vi "Continuous Euler Angles.vi"() -> ()   [LabVIEW 2012]
uses:
  <vilib>/Platform/TimedLoop/XDataNode/timing_clust.ctl
  <vilib>/Platform/TimedLoop/XDataNode/nitl_modes.ctl
  <vilib>/Platform/TimedLoop/XDataNode/wakeup.ctl
  <instrlib>/MicroStrain 3DM-GXx/Public/Data/Parse Message VIs/Parse (Euler Angles).vi
  <vilib>/platform/TimedLoop/XDataNode/XDataNode.xnode
  <instrlib>/MicroStrain 3DM-GXx/MicroStrain 3DM-GXx.lvlib
  <vilib>/Platform/TimedLoop/XDataNode/XDNodeRunTimeDep.lvlib
panel:
  out "Yaw":dbl(graph)
  out "Pitch":dbl(graph)
  out "Roll":dbl(graph)
  out "Euler Angle Timer":u32
  out "Roll, Pitch, Yaw (Degrees)":cluster{dbl, dbl, dbl}(knob) caption="Red Green Blue" scale=-180.0..180.0
  in  "Stop":bool
  in  "VISA resource name":refnum<visa-resource-name>="COM21"
  in  "Measurement Type":u16(ring)=5 items=["Euler Angles"=5]
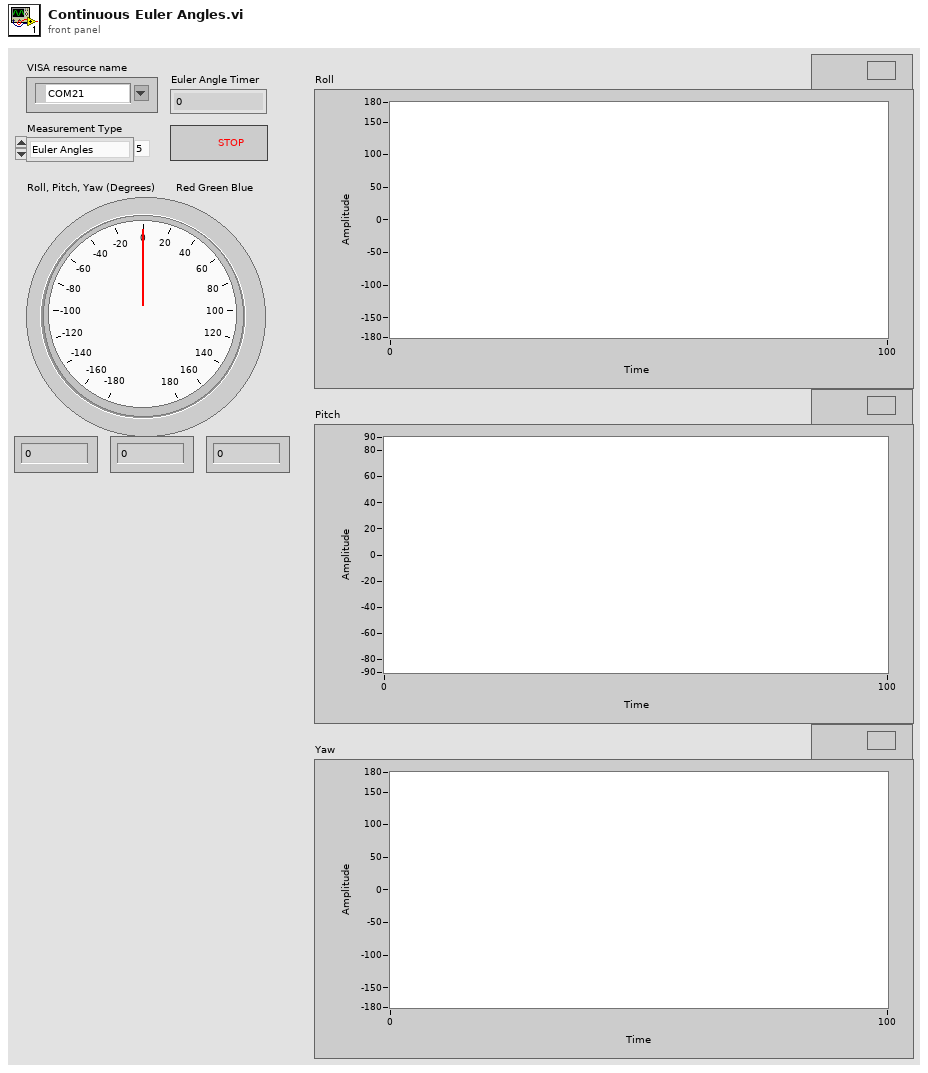
[diagram p1: front panel]
types:
  T1 = typedef "XDNodeRunTimeDep.lvlib/timing_clust.ctl" = cluster{"Expected End [f-1]":u64, "Actual End [f-1]":u64, "Finished Late? [f-1]":bool, "Expected End [i-1]":u64, "Actual End [i-1]":u64, "Finished Late? [i-1]":bool, "Expected Start [i]":u64, "Actual Start [i]":u64, "Expected Start [f]":u64, "Actual Start [f]":u64, "Source Name":string, "Structure Name":string, "Period":i64, "Deadline":i64, "Offset":i64, "Start":i64, "Priority":i32, "Timeout":i32, "Mode":T2, "Wakeup Reason":T3, "Error":errorcluster, "Source Type":string, "Secondary Source Type":string, "Global End Time":u64, "Global Start Time":u64, "Frame Duration":u64, "Iteration Duration":u64, "Assigned CPU":i32, "I/O Scan Engine Mode":u32}
  T2 = typedef "XDNodeRunTimeDep.lvlib/nitl_modes.ctl" = enum32{"No Change", "Process missed periods, maintain original phase", "Discard missed periods, maintain original phase", "Process missed periods, ignore original phase", "Discard missed periods, ignore original phase"}
  T3 = typedef "XDNodeRunTimeDep.lvlib/wakeup.ctl" = enum32{"Normal", "Aborted", "Asynchronous wakeup", "Timing source error", "Timed loop error", "Timeout"}
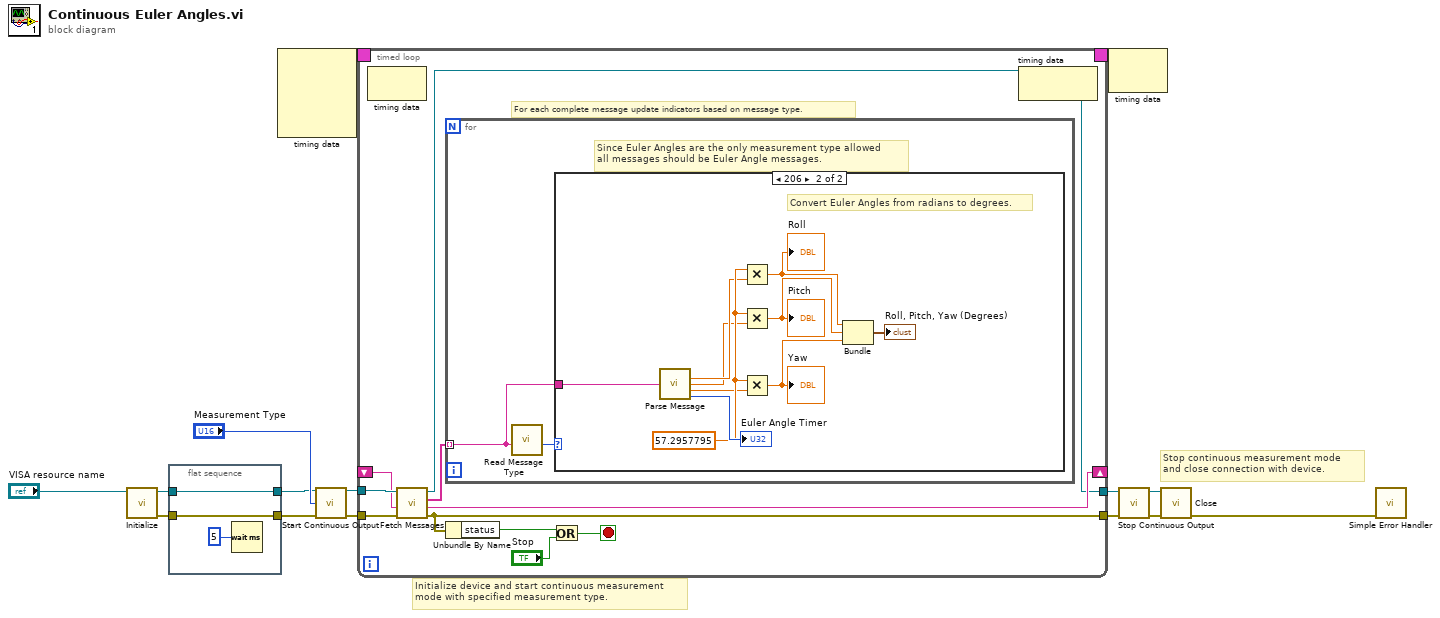
[diagram p0: block diagram]
diagram:
  # "Stop continuous measurement mode \nand close connection with device."
  # "Initialize device and start continuous measurement \nmode with specified measurement type."
  n1 = call "Initialize.vi"("VISA resource name"="VISA resource name") -> ("error out"=w5:errorcluster, "VISA resource name out"=w3:refnum<visa-resource-name>)  [unwired: 9 in]
  n2 = flat-sequence {
    tunnel: [w17] -> w6
    tunnel: w5 -> [w17]
    tunnel: [w16] -> w4
    tunnel: w3 -> [w16]
    frame #0 {
      n3 = Wait (ms)(milliseconds to wait=u32 5) -> ()  [unwired: 1 out]
    }
  }
  n4 = node-c288() -> (w2:T1)  [unwired: 4 in]
  n5 = call <instrlib>:"Start Continuous Output.vi"("VISA resource name"=w4, "Continuous Measurement Type (Raw Accelerometer and Angular Rate)"="Measurement Type", "error in (no error)"=w6) -> ("VISA resource name out"=w13:refnum<visa-resource-name>, "error out"=w12:errorcluster)  [unwired: 11 in]
  n6 = timed-loop {
    tunnel: w13 -> [w28]
    tunnel: w12 -> [w27]
    shift-right: [w25] -> _
    shift-left: _ -> [w26]
    tunnel: [w23] -> w11
    tunnel: [w22] -> w10
    timing: w2 -> [_]
    timing-out: [_] -> w1
    stop <- w19 stop-if-true
    # "For each complete message update indicators based on message type."
    n7 = node-c288() -> ()  [unwired: 1 in, 1 out]
    n8 = call <instrlib>:"Fetch Messages.vi"("error in (no error)"=w27, "Remainder In"=w26, "VISA resource name"=w28) -> ("error out"=w22:errorcluster, "Remainder Out"=w25:string, "Complete Messages"=w24:string[], "VISA resource name out"=w23:refnum<visa-resource-name>)  [unwired: 5 in]
    n9 = for {
      tunnel: w24 -> [w31] mode=indexing
      # "Since Euler Angles are the only measurement type allowed \nall messages should be Euler Angle messages."
      n10 = call <instrlib>:"Read Message Type.vi"("Message"=w31) -> ("Ring"=w32:u16)  [unwired: 10 in]
      n11 = case shown="206" w32 {
        tunnel: w31 -> [_ w42]
        frame 0, Default {
        }
        frame 206 {
          w40 = 57.2957795 ("x")
          # "Convert Euler Angles from radians to degrees."
          n12 = call-poly <instrlib>:"Parse Message.vi"("Message In"=w42) -> ("Roll"=w39:sgl, "Pitch"=w38:sgl, "Yaw"=w37:sgl, "Timer"=→"Euler Angle Timer":u32)  [unwired: 11 in]
          n13 = Multiply(x=w40, y=w39) -> (x*y=w35:dbl)
          "Roll" <- w35
          n14 = Multiply(x=w40, y=w38) -> (x*y=w34:dbl)
          "Pitch" <- w34
          n15 = Multiply(x=w40, y=w37) -> (x*y=w33:dbl)
          "Yaw" <- w33
          n16 = Bundle(w35, w34, w33) -> (→"Roll, Pitch, Yaw (Degrees)":cluster{dbl, dbl, dbl})  [unwired: 1 in]
        }
      }
    }
    n17 = Unbundle By Name(w22) -> ("status"=w21:bool)
    n18 = Or(x=w21, y="Stop") -> (x .or. y?=w19:bool)
    n19 = node-c288() -> ()  [unwired: 1 in, 1 out]
  }
  n20 = node-c288(w1) -> ()  [unwired: 1 out]
  n21 = call <instrlib>:"Stop Continuous Output.vi"("error in (no error)"=w10, "VISA resource name"=w11) -> ("error out"=w9:errorcluster, "VISA resource name out"=w8:refnum<visa-resource-name>)  [unwired: 8 in]
  n22 = call <instrlib>:"Close.vi"("error in (no error)"=w9, "VISA resource name"=w8) -> ("error out"=w7:errorcluster)  [unwired: 9 in]
  n23 = call <vilib>:"Simple Error Handler.vi"("error in (no error)"=w7) -> ()  [unwired: 4 in, 5 out]
